vi "Support Global.vi"() -> ()   [LabVIEW 2021, in "DAQ Hardware.lvlib"]
uses:
  DAQ Hardware.lvlib
  Class/Abstract/Abstract.lvclass
  User Interface/AI Channel Setting.ctl
  DI Channel Setting.ctl
panel:
  in  "DI  Setting":T1
  in  "AI Setting":T2={"Physical Channel"=["6363/ai0", "6363/ai1", "6363/ai2"], "Name to assign"=[], "input terminal configuration"=enum."RSE", "minimum value"=0.0, "maximum value"=10.0, "units"=enum."Volts", "custom scale name"="", "sample mode"=enum."Finite Samples", "rate"=5000.0, "samples per channel"=1000.0} {"rate" format="%#_13g"; "maximum value" format="%#_13g"; "minimum value" format="%#_13g"}
  in  "Abstract.lvclass":refnum<class "Abstract.lvclass">
  in  "DAQ Type":enum16{"Hardware", "Simulation"}(ring)
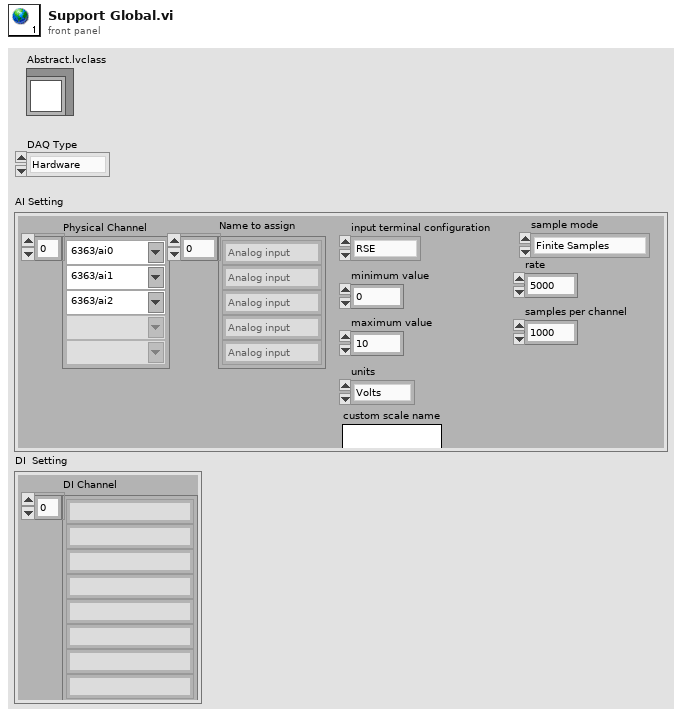
[diagram p1: front panel]
types:
  T1 = typedef "DAQ Hardware.lvlib/DI Channel Setting.ctl" = cluster{"DI Channel":string[]}
  T2 = typedef "DAQ Hardware.lvlib/AI Channel Setting.ctl" = cluster{"Physical Channel":string[], "Name to assign":string[], "input terminal configuration":enum16{"RSE", "NRSE", "Differential"}, "minimum value":dbl, "maximum value":dbl, "units":enum16{"Volts"}, "custom scale name":string, "sample mode":enum16{"Finite Samples", "Continuous Samples", "Hardware Timed Single Point"}, "rate":dbl, "samples per channel":dbl}
diagram:
